vi "Main.vi"() -> ()   [LabVIEW 2024]
uses:
  40054479-b80a-4381-ad9d-7fff89c46ed6.vi
  8d61351b-f6e0-4b92-a084-70b812052fdc.vi
  8cda92f2-d50d-441a-9ff2-4cbea2f9377b.vi
  d4b91904-d550-4aeb-ba5d-fe1c18ee7e5f.vi
panel:
  out "Error Out":errorcluster
  in  "Launch VIs via ...":T1(ring)
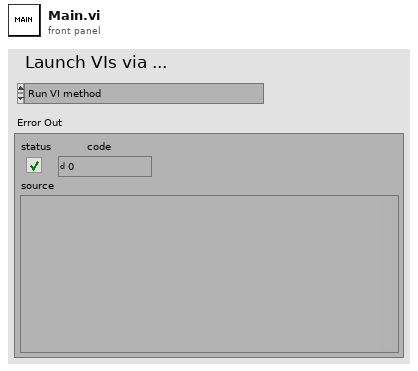
[diagram p1: front panel]
types:
  T1 = enum16{"Run VI method", "Asynchronous Call By Reference node"}
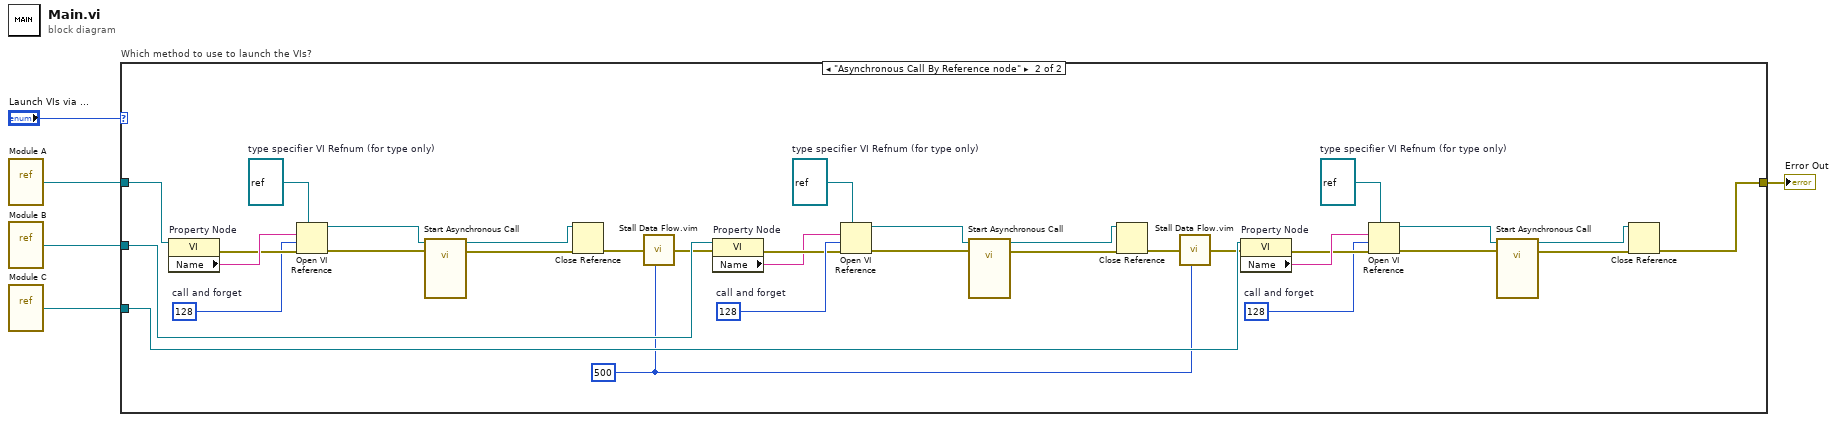
[diagram p0: block diagram]
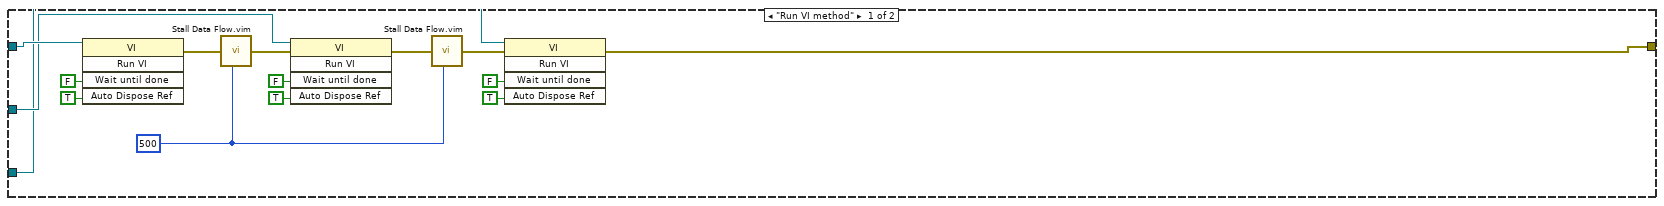
[diagram p2: hidden frame]
diagram:
  n1 = vi-ref "Module A.vi"() -> (w4:refnum<vi>)
  n2 = vi-ref "Module B.vi"() -> (w3:refnum<vi>)
  n3 = vi-ref "Module C.vi"() -> (w2:refnum<vi>)
  n4 = case "Which method to use to launch the VIs?" shown="\"Asynchronous Call By Reference node\"" "Launch VIs via ..." {
    tunnel: w4 -> [w18 w45]
    tunnel: w3 -> [w14 w35]
    tunnel: w2 -> [w10 w25]
    tunnel: [w6 w24] -> w1
    frame "Run VI method" {
      w7 = u32 500 ("milliseconds to wait")
      n5 = invoke class="VI" method="Run VI"(reference=w18, "Wait until done"=FALSE ("Wait Until Done"), "Auto Dispose Ref"=TRUE ("Auto Dispose Reference")) -> (error out=w15:errorcluster)  [unwired: 2 in, 4 out]
      n6 = call "Stall Data Flow.vim"("value in"=w15, "milliseconds to wait"=w7) -> ("value out"=w9:errorcluster)  [unwired: 1 out]
      n7 = invoke class="VI" method="Run VI"(reference=w14, error in=w9, "Wait until done"=FALSE ("Wait Until Done"), "Auto Dispose Ref"=TRUE ("Auto Dispose Reference")) -> (error out=w11:errorcluster)  [unwired: 1 in, 4 out]
      n8 = call "Stall Data Flow.vim"("value in"=w11, "milliseconds to wait"=w7) -> ("value out"=w8:errorcluster)  [unwired: 1 out]
      n9 = invoke class="VI" method="Run VI"(reference=w10, error in=w8, "Wait until done"=FALSE ("Wait Until Done"), "Auto Dispose Ref"=TRUE ("Auto Dispose Reference")) -> (error out=w6:errorcluster)  [unwired: 1 in, 4 out]
    }
    frame "Asynchronous Call By Reference node" {
      w21 = u32 500 ("milliseconds to wait")
      w28 = refnum<vi> refnum  # type specifier VI Refnum (for type only)
      w27 = 128  # call and forget
      w43 = refnum<vi> refnum  # type specifier VI Refnum (for type only)
      w44 = 128  # call and forget
      w47 = refnum<vi> refnum  # type specifier VI Refnum (for type only)
      w46 = 128  # call and forget
      n10 = property on="Property Node" class="VI"(reference=w45) -> (error out=w48:errorcluster, "Name"=w49:string)  [unwired: 1 in, 1 out]
      n11 = Open VI Reference(type specifier VI Refnum (for type only)=w47, vi path=w49, options=w46, error in (no error)=w48) -> (vi reference=w50:refnum<vi>, error out=w52:errorcluster)  [unwired: 2 in]
      n12 = call-by-ref "Start Asynchronous Call"(reference=w50, error in=w52) -> (reference out=w53:refnum<vi>, error out=w51:errorcluster)  [unwired: 11 in, 1 out]
      n13 = Close Reference(reference=w53, error in (no error)=w51) -> (error out=w36:errorcluster)
      n14 = call "Stall Data Flow.vim"("value in"=w36, "milliseconds to wait"=w21) -> ("value out"=w23:errorcluster)  [unwired: 1 out]
      n15 = property on="Property Node" class="VI"(reference=w35, error in=w23) -> (error out=w42:errorcluster, "Name"=w41:string)  [unwired: 1 out]
      n16 = Open VI Reference(type specifier VI Refnum (for type only)=w43, vi path=w41, options=w44, error in (no error)=w42) -> (vi reference=w40:refnum<vi>, error out=w38:errorcluster)  [unwired: 2 in]
      n17 = call-by-ref "Start Asynchronous Call"(reference=w40, error in=w38) -> (reference out=w37:refnum<vi>, error out=w39:errorcluster)  [unwired: 11 in, 1 out]
      n18 = Close Reference(reference=w37, error in (no error)=w39) -> (error out=w26:errorcluster)
      n19 = call "Stall Data Flow.vim"("value in"=w26, "milliseconds to wait"=w21) -> ("value out"=w22:errorcluster)  [unwired: 1 out]
      n20 = property on="Property Node" class="VI"(reference=w25, error in=w22) -> (error out=w29:errorcluster, "Name"=w30:string)  [unwired: 1 out]
      n21 = Open VI Reference(type specifier VI Refnum (for type only)=w28, vi path=w30, options=w27, error in (no error)=w29) -> (vi reference=w31:refnum<vi>, error out=w33:errorcluster)  [unwired: 2 in]
      n22 = call-by-ref "Start Asynchronous Call"(reference=w31, error in=w33) -> (reference out=w34:refnum<vi>, error out=w32:errorcluster)  [unwired: 11 in, 1 out]
      n23 = Close Reference(reference=w34, error in (no error)=w32) -> (error out=w24:errorcluster)
    }
  }
  "Error Out" <- w1
